vi "Data to Single Line String_Do.vi"(8 "error in (no error)":errorcluster, 11 "Report Data in":refnum<class "Report Data.lvclass">) -> (0 "error out":errorcluster, 3 "String Data":string)   [LabVIEW 2020, in "ProjectBuilder.lvlib" / "Report Data.lvclass"]
doc: "Format private data into a string.\n\nThe default implementation created the following string:\n[Start Time] Action name: [Success or Failed (code)]"
uses:
  Report Data.lvclass
  Report Data.lvclass/Report Data.ctl
  ProjectBuilder.lvlib
  PPL/HDH.ClassLoader.lvlibp
  Project Action/Project Action.lvclass
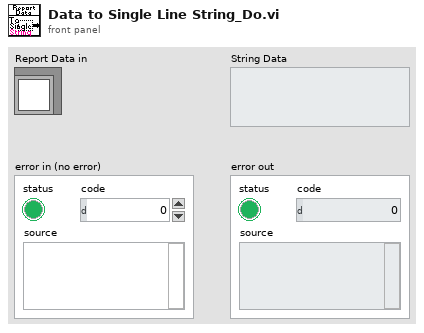
[diagram p1: front panel]
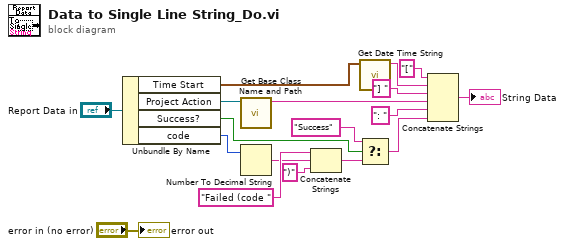
[diagram p0: block diagram]
diagram:
  n1 = Unbundle By Name("Report Data in") -> ("Time Start"=w16:timestamp, "Project Action"=w3:refnum<class "Project Action.lvclass">, "Success?"=w11:bool, "code"=w9:i32)
  n2 = call "Get Base Class Name and Path.vi"("Class"=w3) -> ("Base Class Name"=w2:string)  [unwired: 8 in, 2 out]
  n3 = Number To Decimal String(number=w9) -> (decimal integer string=w7:string)  [unwired: 1 in]
  n4 = Concatenate Strings("Failed (code ", w7, ")" ("string")) -> (w5:string)
  n5 = call "Get Date Time String.vi"("Time (Current time)"=w16) -> ("Time String"=w14:string)  [unwired: 10 in]
  n6 = Select(t="Success", s=w11, f=w5) -> (s? t:f=w4:string)
  n7 = Concatenate Strings("[" ("string"), w14, "] " ("string"), w2, ": " ("string"), w4) -> (→"String Data":string)
  "error out" <- "error in (no error)"
